vi "Update CD Channel Tree.vi"(7 "CD List":refnum<vi>, 8 "error in (no error)":errorcluster, 11 "Channel Array":refnum<class "ChannelVS.lvclass">[](array[class])) -> (0 "error out":errorcluster)   [LabVIEW 2020, in "Shared Variables CD 2.0 Configuration.lvlib"]
uses:
  Shared Variables CD 2.0 Configuration.lvlib
  ChannelVS/ChannelVS.lvclass
  built/windows/Channel.lvlibp/Channel.lvclass
  C:/Users/Administrator/Desktop/GIT/Shared-Variable-Custom-Device-2.0/Source/built/windows/Channel.lvlibp/Channel.lvclass
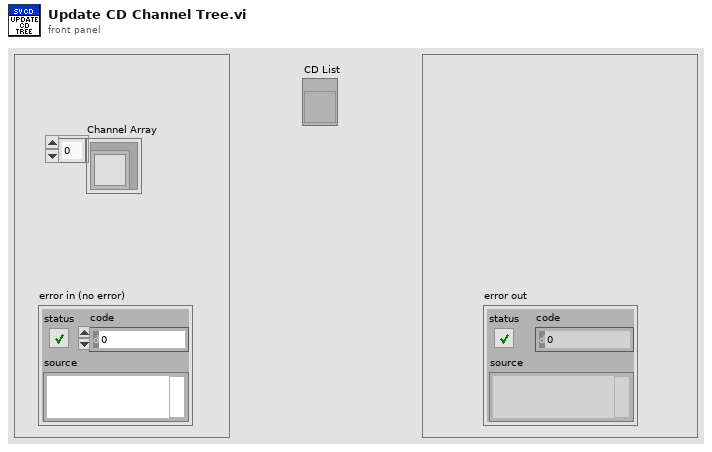
[diagram p1: front panel]
types:
  T1 = typedef "Channel.lvlibp/NI_Data Type.lvlib/Data Type.ctl" = enum8{"Invalid Type", "Void", "I8", "I16", "I32", "I64", "U8", "U16", "U32", "U64", "Single Float", "Double Float", "Extended Float", "Single Complex", "Double Complex", "Extended Complex", "Enum U8", "Enum U16", "Enum U32", "Enum U64", "Single Float With Unit", "Double Float With Unit", "Extended Float With Unit", "Single Complex with Unit", "Double Complex with Unit", "Extended Complex with Unit", "Boolean", "String", "Path", "Picture", "Tag", "Array", "Cluster", "Variant", "LV Variant", "Waveform", "Timestamp", "Digital Waveform", "Digital Data", "ExpressData", "Refnum", "External Data", "VI", "Poly VI", "LabVIEW Class Instance", "Fixed Point", "Set Collection", "Map Collection"}
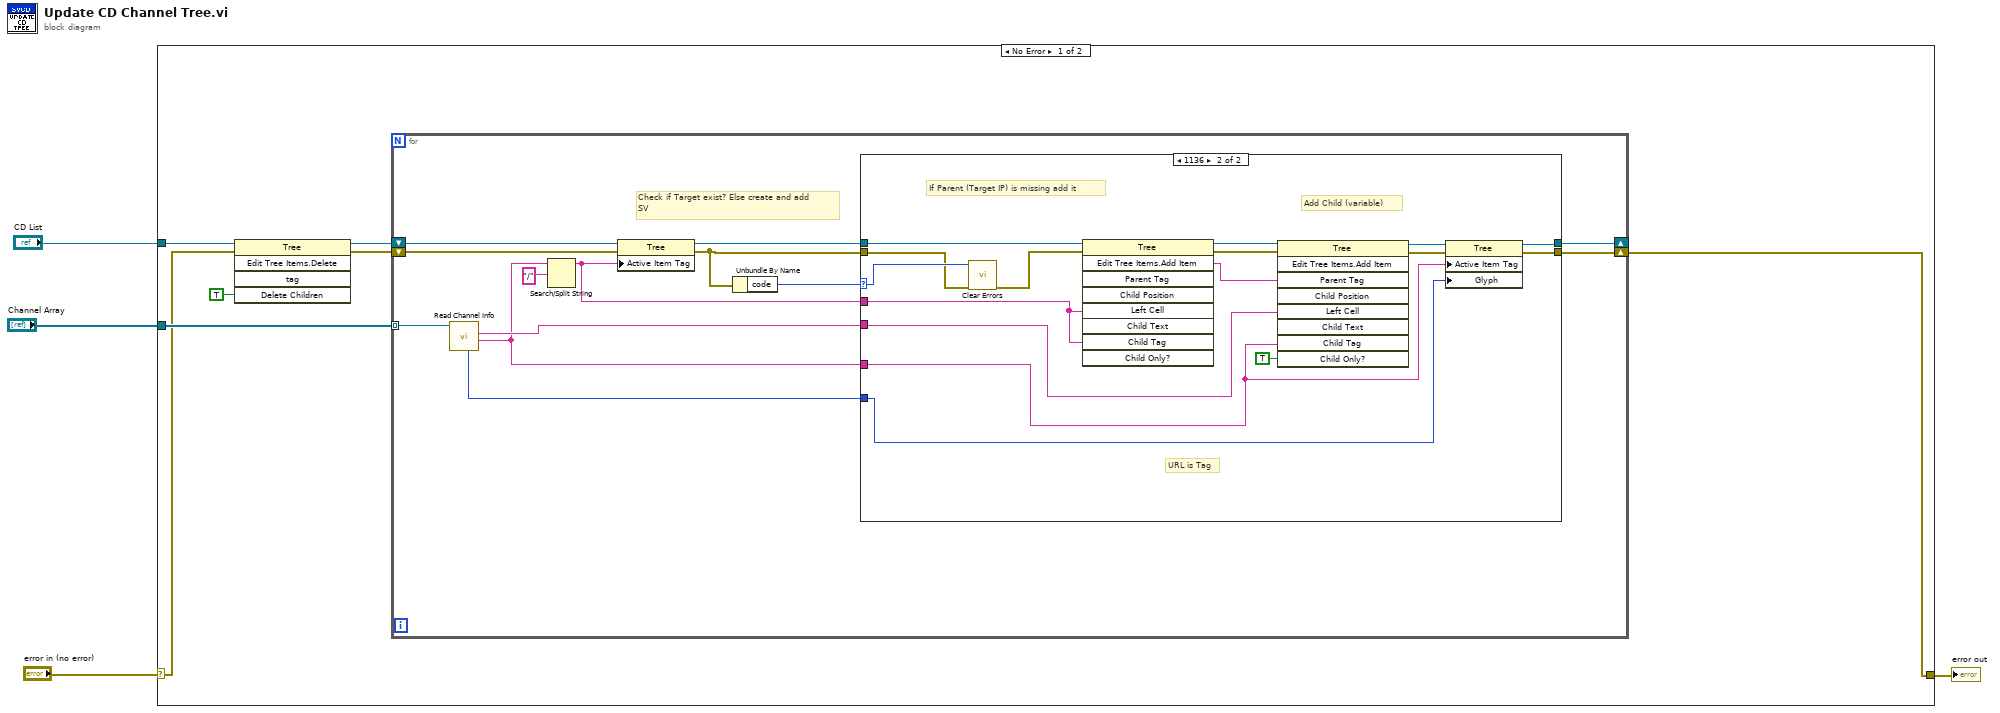
[diagram p0: block diagram]
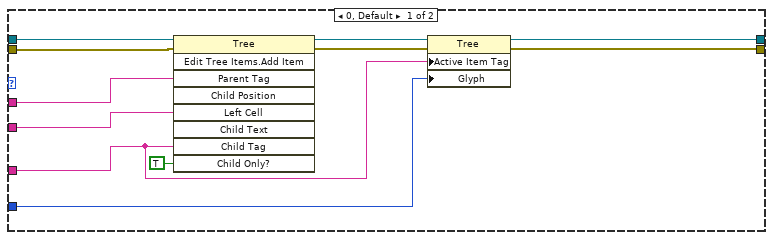
[diagram p2: hidden frame]
diagram:
  n1 = case shown="No Error" "error in (no error)" {
    selector: "error in (no error)" -> [w7 w52]
    tunnel: "CD List" -> [w8 _]
    tunnel: "Channel Array" -> [w11 _]
    tunnel: [w10 w52] -> w1
    frame No Error {
      n2 = invoke class="Tree" method="Edit Tree Items.Delete"(reference=w8, error in=w7, "Delete Children"=TRUE ("Delete Children?")) -> (reference out=w5:refnum<vi>, error out=w6:errorcluster)  [unwired: 2 in, 3 out]
      n3 = for {
        tunnel: w11 -> [w13] mode=indexing
        shift-right: [w19] -> w10
        shift-left: w6 -> [w16]
        shift-right: [w18] -> _
        shift-left: w5 -> [w17]
        # "Check if Target exist? Else create and add\nSV"
        n4 = call "Read Channel Info.vi"("Channel in"=w13) -> ("URL"=w12:string, "Name"=w15:string, "DataType"=w14:T1)  [unwired: 5 in, 3 out]
        n5 = Search/Split String(string=w12, search string/char (-)="/") -> (substring before match=w23:string)  [unwired: 1 in, 2 out]
        n6 = property on="Property Node" class="Tree"(reference=w17, error in=w16, "Active Item Tag"=w23) -> (reference out=w21:refnum<vi>, error out=w20:errorcluster)
        n7 = Unbundle By Name(w20) -> ("code"=w22:i32)
        n8 = case shown="1136" w22 {
          selector: w22 -> [_ w45]
          tunnel: w15 -> [w35 w46]
          tunnel: w12 -> [w27 w38]
          tunnel: w23 -> [w34 w50]
          tunnel: w21 -> [w33 w51]
          tunnel: w20 -> [w32 w44]
          tunnel: [w28 w39] -> w19
          tunnel: w14 -> [w26 w37]
          tunnel: [w30 w41] -> w18
          frame 0, Default {
            n9 = invoke on="Invoke Node" class="Tree" method="Edit Tree Items.Add Item"(reference=w33, error in=w32, "Parent Tag"=w34, "Left Cell"=w35, "Child Tag"=w27, "Child Only?"=TRUE) -> (reference out=w31:refnum<vi>, error out=w29:errorcluster)  [unwired: 3 in, 7 out]
            n10 = property class="Tree"(reference=w31, error in=w29, "Active Item Tag"=w27, "Glyph"=w26) -> (reference out=w30:refnum<vi>, error out=w28:errorcluster)
          }
          frame 1136 {
            # "Add Child (variable)"
            # "If Parent (Target IP) is missing add it"
            # "URL is Tag"
            n11 = call <vilib>:"Clear Errors.vi"("error in (no error)"=w44, "specific error code to clear (0: all)"=w45) -> ("error out"=w43:errorcluster)  [unwired: 4 in, 1 out]
            n12 = invoke class="Tree" method="Edit Tree Items.Add Item"(reference=w51, error in=w43, "Left Cell"=w50, "Child Tag"=w50) -> (reference out=w49:refnum<vi>, error out=w48:errorcluster, "Edit Tree Items:Add Item"=w47:string)  [unwired: 5 in, 6 out]
            n13 = invoke on="Invoke Node" class="Tree" method="Edit Tree Items.Add Item"(reference=w49, error in=w48, "Parent Tag"=w47, "Left Cell"=w46, "Child Tag"=w38, "Child Only?"=TRUE) -> (reference out=w42:refnum<vi>, error out=w40:errorcluster)  [unwired: 3 in, 7 out]
            n14 = property class="Tree"(reference=w42, error in=w40, "Active Item Tag"=w38, "Glyph"=w37) -> (reference out=w41:refnum<vi>, error out=w39:errorcluster)
          }
        }
      }
    }
    frame Error {
    }
  }
  "error out" <- w1
